vi "MListbox Move Selected Up.vi"(8 "error in (no error)":errorcluster, 11 "Multicolumn ListBox in":refnum<class "Multicolumn ListBox.lvclass">) -> (0 "error out":errorcluster, 3 "Multicolumn ListBox out":refnum<class "Multicolumn ListBox.lvclass">)   [LabVIEW 2012, in "Multicolumn ListBox.lvclass"]
uses:
  Multicolumn ListBox.lvclass
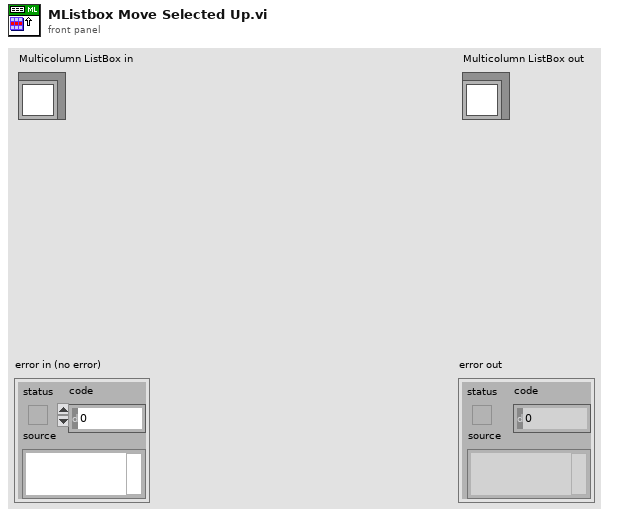
[diagram p1: front panel]
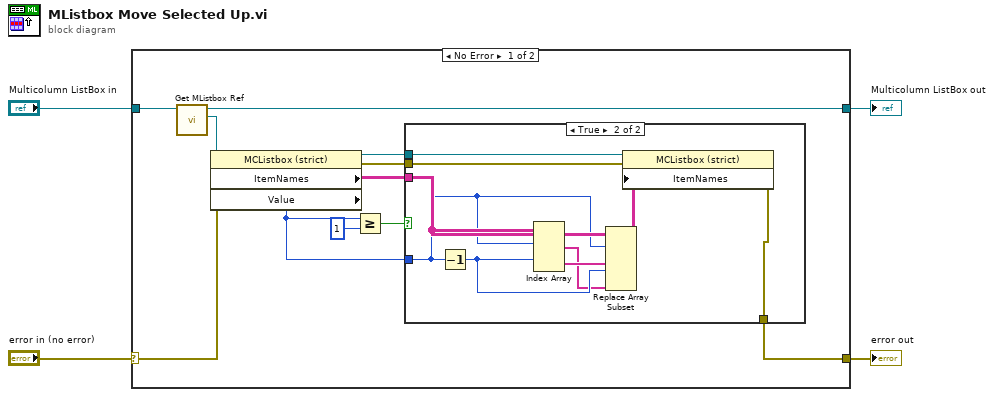
[diagram p0: block diagram]
diagram:
  n1 = case shown="No Error" "error in (no error)" {
    selector: "error in (no error)" -> [w10 w27]
    tunnel: [w9 w27] -> w3
    tunnel: [w14 w26] -> w1
    tunnel: "Multicolumn ListBox in" -> [w15 w26]
    frame No Error {
      n2 = call "Get MListbox Ref.vi"("Multicolumn ListBox in"=w15) -> ("MListbox Ref"=w13:refnum<vi>, "Multicolumn ListBox out"=w14:refnum<class "Multicolumn ListBox.lvclass">)  [unwired: 8 in, 1 out]
      n3 = property class="MCListbox (strict)"(reference=w13, error in=w10) -> (reference out=w12:refnum<vi>, error out=w11:errorcluster, "ItemNames"=w8:string[][], "Value"=w7:i32)
      n4 = Greater Or Equal?(x=w7, y=1 ("x")) -> (x >= y?=w6:bool)
      n5 = case shown="True" w6 {
        tunnel: w12 -> [_ w25]
        tunnel: w11 -> [w16 w24]
        tunnel: [w16 w23] -> w9
        tunnel: w8 -> [_ w22]
        tunnel: w7 -> [_ w17]
        frame False {
        }
        frame True {
          n6 = Decrement(x=w17) -> (x-1=w20:i32)
          n7 = Index Array(array=w22, index (row) #1=w17, index (row) #2=w20) -> (element #1=w19:string[], element #2=w21:string[])  [unwired: 2 in]
          n8 = Replace Array Subset(array=w22, new element #1=w21, index (row) #1=w17, new element #2=w19, index (row) #2=w20) -> (w18:string[][])  [unwired: 2 in]
          n9 = property class="MCListbox (strict)"(reference=w25, error in=w24, "ItemNames"=w18) -> (error out=w23:errorcluster)  [unwired: 1 out]
        }
      }
    }
    frame Error {
    }
  }
  "error out" <- w3
  "Multicolumn ListBox out" <- w1
